vi "GC Vacuum - Step 4.vi"(7 "Step":i32, 8 "error in":errorcluster, 9 "Test Results In":T8, 10 "Gas":T1, 11 "GC Configuration":T2) -> (0 "error out":errorcluster, 1 "Test Results Out":T8, 2 "Gas Out":T1 caption="Gas", 3 "GC Configuration Out":T2)   [LabVIEW 2015]
uses:
  Controls/Test Information.ctl
  Controls/Vacuum Test.ctl
  Controls/Test Timing.ctl
  Controls/Vaccum Thresholds.ctl
  Controls/Helium Test.ctl
  Controls/Helium Thresholds.ctl
  CAN Communication/Gas/Typedefs/Session Handle.ctl
  CAN Communication/Gas/Gas.lvclass
  Controls/Test Results.ctl
  Controls/Step Result.ctl
  CAN Communication/Gas/Typedefs/Valves.ctl
  SubVIs/Timing/Timing.lvlib
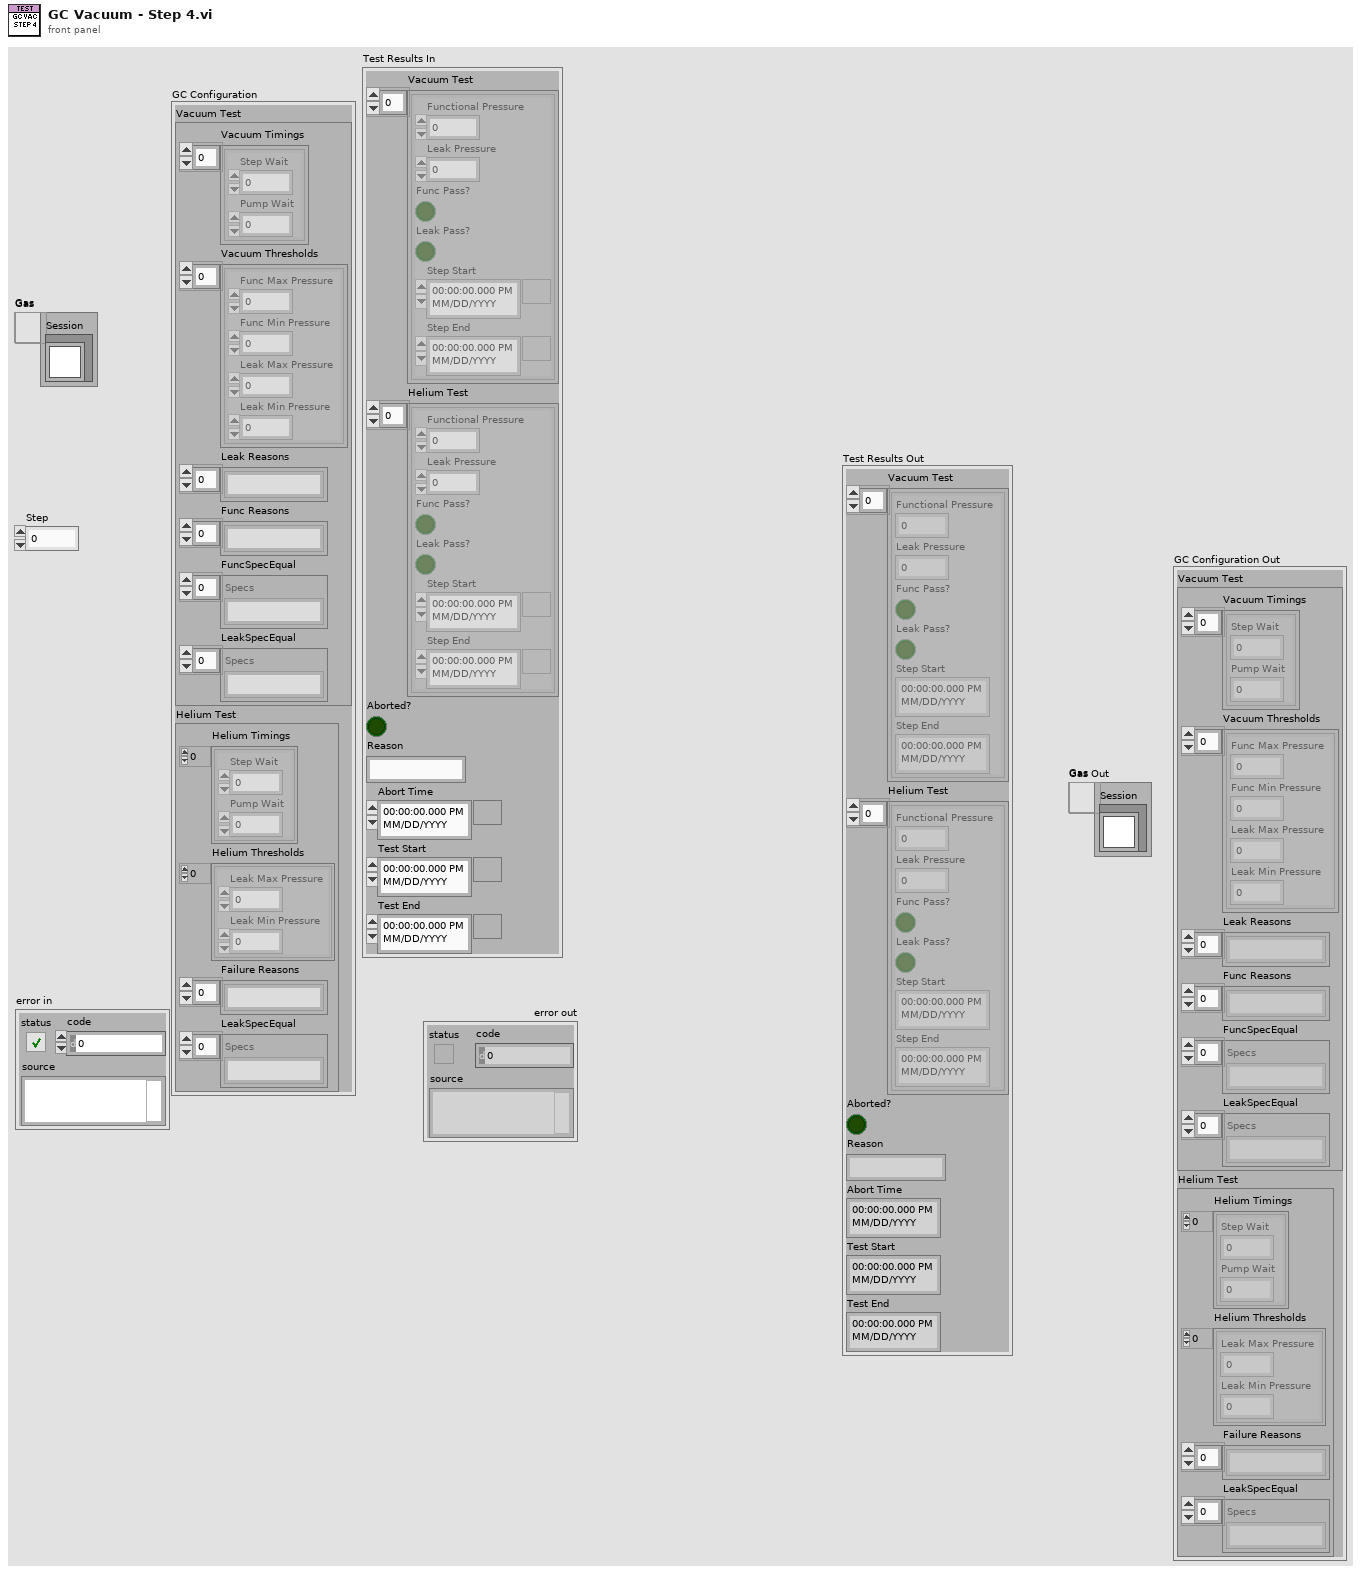
[diagram p1: front panel]
types:
  T1 = typedef "Gas.lvclass/Session Handle.ctl" = refnum<data-value>
  T2 = typedef "Test Information.ctl" = cluster{"Vacuum Test":T3, "Helium Test":T6}
  T3 = typedef "Vacuum Test.ctl" = cluster{"Vacuum Timings":T4[], "Vacuum Thresholds":T5[], "Leak Reasons":string[], "Func Reasons":string[], "FuncSpecEqual":string[], "LeakSpecEqual":string[]}
  T4 = typedef "Test Timing.ctl" = cluster{"Step Wait":dbl, "Pump Wait":dbl}
  T5 = typedef "Vaccum Thresholds.ctl" = cluster{"Func Max Pressure":dbl, "Func Min Pressure":dbl, "Leak Max Pressure":dbl, "Leak Min Pressure":dbl}
  T6 = typedef "Helium Test.ctl" = cluster{"Helium Timings":T4[], "Helium Thresholds":T7[], "Failure Reasons":string[], "LeakSpecEqual":string[]}
  T7 = typedef "Helium Thresholds.ctl" = cluster{"Leak Max Pressure":dbl, "Leak Min Pressure":dbl}
  T8 = typedef "Test Results.ctl" = cluster{"Vacuum Test":T9[], "Helium Test":T9[], "Aborted?":bool, "Reason":string, "Abort Time":timestamp, "Test Start":timestamp, "Test End":timestamp}
  T9 = typedef "Step Result.ctl" = cluster{"Functional Pressure":dbl, "Leak Pressure":dbl, "Func Pass?":bool, "Leak Pass?":bool, "Step Start":timestamp, "Step End":timestamp}
  T10 = typedef "Gas.lvclass/Valves.ctl" = u16
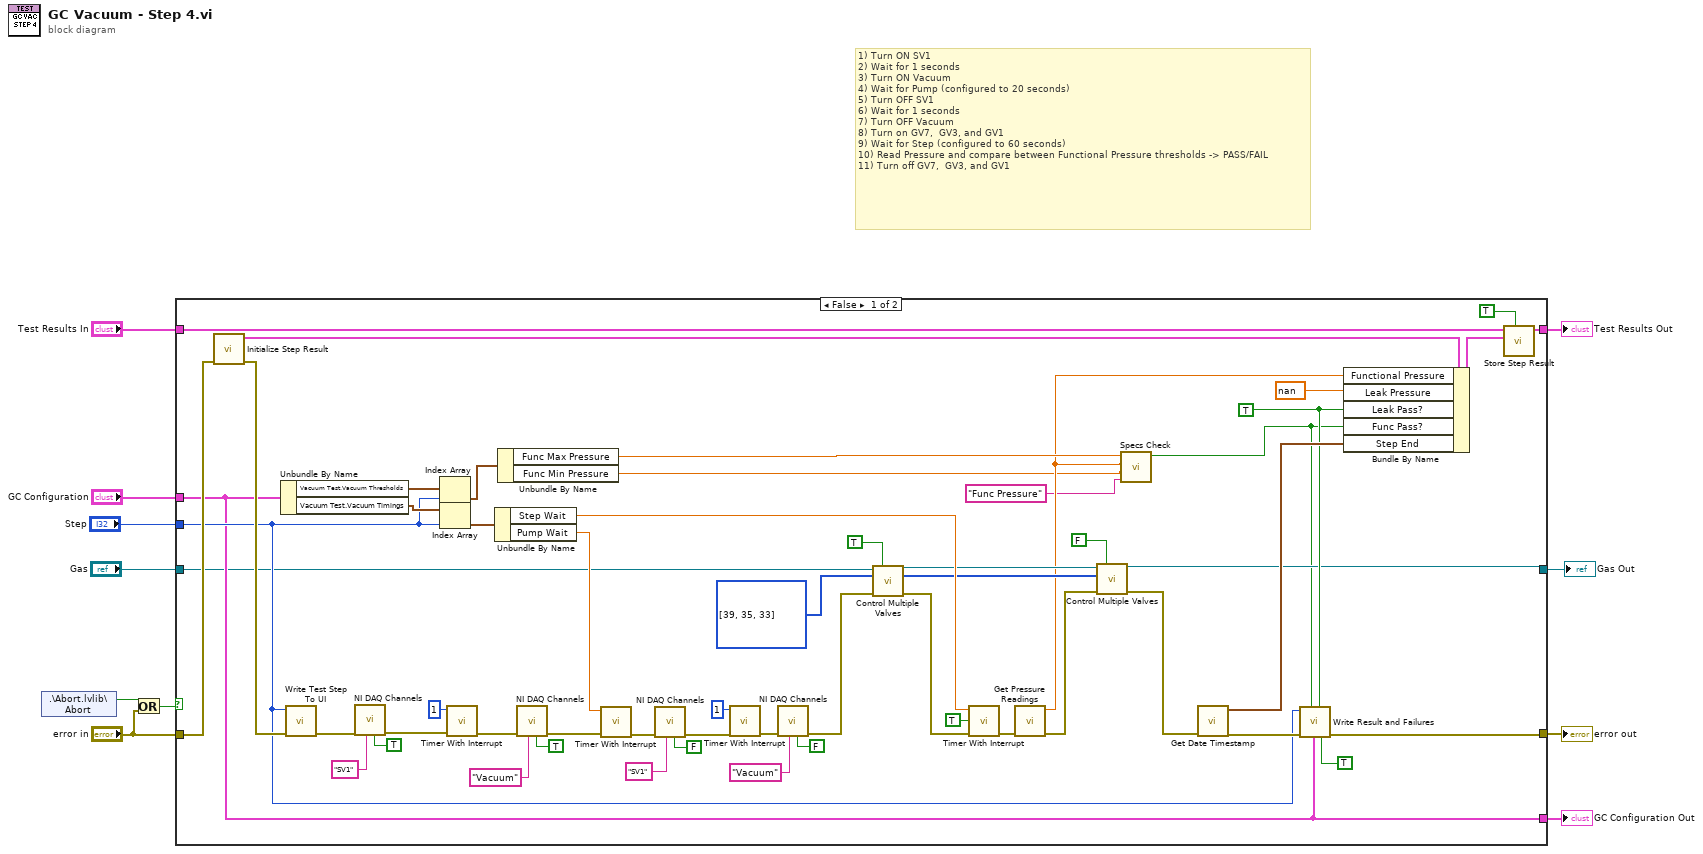
[diagram p0: block diagram]
diagram:
  # "1) Turn ON SV1\n2) Wait for 1 seconds\n3) Turn ON Vacuum\n4) Wait for Pump (configured to 20 seconds)\n5) Turn OFF SV1\n6) Wait for 1 seconds\n7) Turn OFF Vacuum\n8) Turn on GV7,  GV3, and GV1\n9) Wait for Step (configured to 60 seconds)\n10) Read Pressure and compare between Functional Pressure thresholds -> PASS/FAIL\n11) Turn off GV7,  GV3, and GV1"
  n1 = shared-variable ".\\Abort.lvlib\\Abort"() -> (w10:bool)  [unwired: 1 in, 1 out]
  n2 = Or(x=w10, y="error in") -> (x .or. y?=w9:bool)
  n3 = case shown="False" w9 {
    tunnel: "error in" -> [w67 w70]
    tunnel: "Test Results In" -> [w64 w71]
    tunnel: [w65 w71] -> w7
    tunnel: [w52 w70] -> w6
    tunnel: "GC Configuration" -> [w50 w69]
    tunnel: "Step" -> [w51 _]
    tunnel: [w50 w69] -> w3
    tunnel: [w36 w68] -> w1
    tunnel: "Gas" -> [w44 w68]
    frame False {
      w43 = T10[] [39, 35, 33] items=["GV1"=33, "GV2"=34, "GV3"=35, "GV4"=36, "GV5"=37, "GV6"=38, "GV7"=39, "GV8"=40, "GV9"=41, "GV10"=42, "GV11"=43, "LV3"=51, "LV4"=52] ("Valves")
      w46 = TRUE ("Leak Pass?")
      n4 = call "Initialize Step Result.vi"("error in (no error)"=w67) -> ("error out"=w66:errorcluster, "New Step Result"=w63:T9)  [unwired: 8 in, 1 out]
      n5 = Unbundle By Name(w50) -> ("Vacuum Test.Vacuum Thresholds"=w60:T5[], "Vacuum Test.Vacuum Timings"=w59:T4[])
      n6 = call "Write Test Step To UI.vi"("error in (no error)"=w66, "Step"=w51) -> ("error out"=w32:errorcluster)  [unwired: 9 in]
      n7 = call "NI DAQ Channels.vi"("Control"=TRUE ("State"), "Channel"="SV1", "error in (no error)"=w32) -> ("error out"=w31:errorcluster)  [unwired: 7 in, 1 out]
      n8 = Index Array(array=w60, index=w51) -> (element=w57:T5)
      n9 = Index Array(array=w59, index=w51) -> (element=w58:T4)
      n10 = call "Timer With Interrupt.vi"("error in (no error)"=w31, "Wait (s)"=1) -> ("error out"=w29:errorcluster)  [unwired: 7 in, 2 out]
      n11 = Unbundle By Name(w58) -> ("Step Wait"=w56:dbl, "Pump Wait"=w48:dbl)
      n12 = Unbundle By Name(w57) -> ("Func Max Pressure"=w15:dbl, "Func Min Pressure"=w13:dbl)
      n13 = call "NI DAQ Channels.vi"("Control"=TRUE ("State"), "Channel"="Vacuum", "error in (no error)"=w29) -> ("error out"=w28:errorcluster)  [unwired: 7 in, 1 out]
      n14 = call "Timer With Interrupt.vi"("error in (no error)"=w28, "Wait (s)"=w48) -> ("error out"=w26:errorcluster)  [unwired: 7 in, 2 out]
      n15 = call "NI DAQ Channels.vi"("Control"=FALSE ("State"), "Channel"="SV1", "error in (no error)"=w26) -> ("error out"=w25:errorcluster)  [unwired: 7 in, 1 out]
      n16 = call "Timer With Interrupt.vi"("error in (no error)"=w25, "Wait (s)"=1) -> ("error out"=w22:errorcluster)  [unwired: 7 in, 2 out]
      n17 = call "NI DAQ Channels.vi"("Control"=FALSE ("State"), "Channel"="Vacuum", "error in (no error)"=w22) -> ("error out"=w23:errorcluster)  [unwired: 7 in, 1 out]
      n18 = call "Control Multiple Valves.vi"("Session Handle in"=w44, "Energize?"=TRUE, "Valves"=w43, "error in (no error)"=w23) -> ("Session Handle out"=w42:T1, "Valves Out"=w41:T10[], "error out"=w40:errorcluster)  [unwired: 8 in, 1 out]
      n19 = call "Timer With Interrupt.vi"("error in (no error)"=w40, "Update UI?"=TRUE, "Wait (s)"=w56) -> ("error out"=w54:errorcluster)  [unwired: 6 in, 2 out]
      n20 = call "Get Pressure Readings.vi"("error in (no error)"=w54) -> ("error out"=w39:errorcluster, "NI-DAQ Pressure"=w14:dbl)  [unwired: 6 in, 3 out]
      n21 = call "Control Multiple Valves.vi"("Session Handle in"=w42, "Energize?"=FALSE, "Valves"=w41, "error in (no error)"=w39) -> ("Session Handle out"=w36:T1, "error out"=w35:errorcluster)  [unwired: 8 in, 2 out]
      n22 = call "Specs Check.vi"("parameter"="Func Pressure", "lower limit"=w13, "x"=w14, "upper limit"=w15) -> ("In Range?"=w16:bool)  [unwired: 6 in, 1 out]
      n23 = call "Get Date Timestamp.vi"("error in (no error)"=w35) -> ("error out"=w53:errorcluster, "current time"=w61:timestamp)  [unwired: 9 in]
      n24 = call "Write Result and Failures.vi"("Vacuum?"=TRUE, "Leak"=w46, "GC Configuration"=w50, "Func"=w16, "error in (no error)"=w53, "Step"=w51) -> ("error out"=w52:errorcluster)  [unwired: 5 in]
      n25 = Bundle By Name(cluster=w63, "Functional Pressure"=w14, "Leak Pressure"=nan ("Step Pressure"), "Leak Pass?"=w46, "Func Pass?"=w16, "Step End"=w61) -> (w62:T9)
      n26 = call "Store Step Result.vi"("Vacuum?"=TRUE, "Step Result"=w62, "Test Results In"=w64) -> ("Test Results Out"=w65:T8)  [unwired: 8 in]
    }
    frame True {
    }
  }
  "error out" <- w6
  "Test Results Out" <- w7
  "GC Configuration Out" <- w3
  "Gas Out" <- w1
